vi "Cross With Speed Reference (1 Ch).vi"(8 "error in (no error)":errorcluster, 10 "Speed Profile (Positions [s])":sgl[](array[numeric]), 11 "Waveform":waveform(sgl)) -> (0 "error out":errorcluster, 3 "Cross phase [degrees]":cluster{"f0":dbl, "df":dbl, "phase":sgl[]})   [LabVIEW 2017, in "VibrationAnalysisFunctions.lvlib"]
uses:
  <vilib>/addons/InsightCM/Utilities/Analysis/Vibration/VibrationAnalysisFunctions.lvlib
  <vilib>/addons/_NISVFA/_Shared subVIs/Controls/svc_Window [Dual FFT].ctl
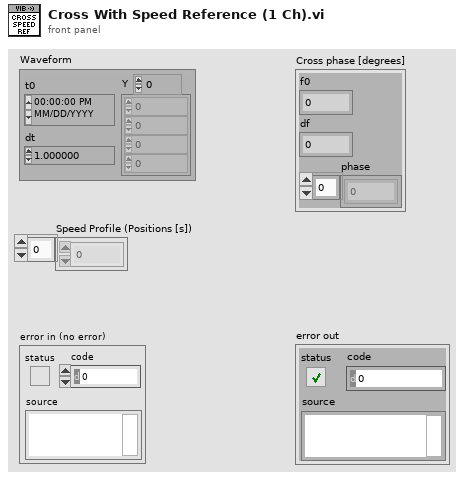
[diagram p1: front panel]
types:
  T1 = cluster{"dB On (T)":bool, "unwrap phase (F)":bool, "convert to degree (T)":bool}
  T2 = typedef "svc_Window [Dual FFT].ctl" = u32
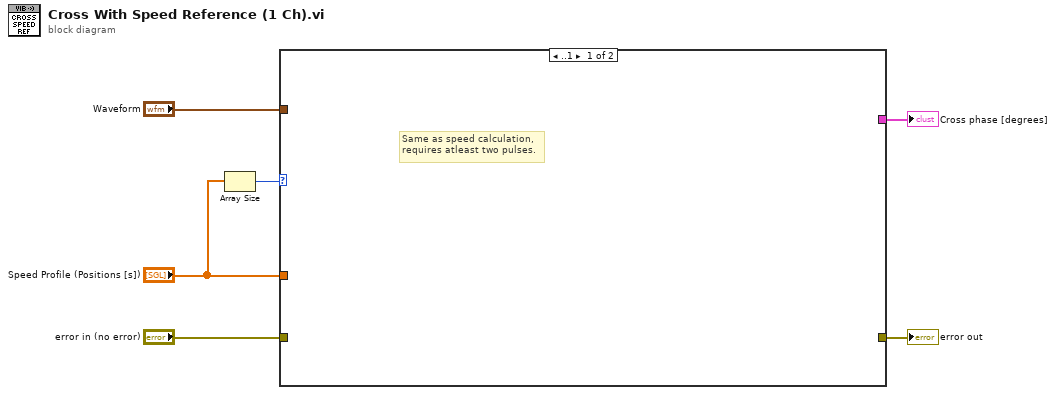
[diagram p0: block diagram]
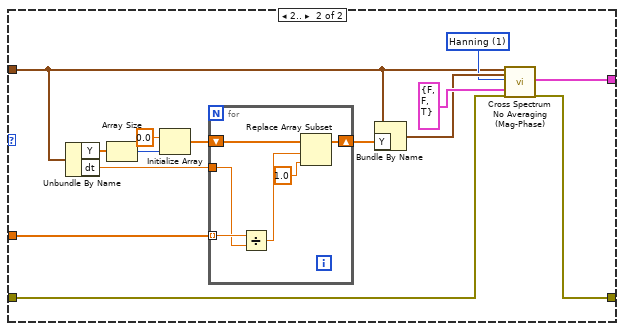
[diagram p2: hidden frame]
diagram:
  n1 = Array Size(array="Speed Profile (Positions [s])") -> (size(s)=w6:i32)
  n2 = case shown="..1" w6 {
    tunnel: "Waveform" -> [_ w7]
    tunnel: "Speed Profile (Positions [s])" -> [_ w8]
    tunnel: [_ w11] -> w3
    tunnel: [_ w9] -> w1
    tunnel: "error in (no error)" -> [_ w10]
    frame ..1 {
      # "Same as speed calculation,\nrequires atleast two pulses."
    }
    frame 2.. {
      w14 = T2 1 items=["None"=0, "Hanning"=1, "Hamming"=2, "Blackman-Harris"=3, "Exact Blackman"=4, "Blackman"=5, "Flat Top"=6, "4 Term B-Harris "=7, "7 Term B-Harris"=8, "Low Sidelobe"=9, "Force - Exponential"=10, "Blackman Nuttall"=11, "Triangle"=30, "Bartlett-Hanning"=31, "Bohman"=32, "Parzen"=33, "Welch"=34, "Kaiser"=60, "Dolph-Chebyshev"=61, "Gaussian"=62] ("window")
      n3 = Unbundle By Name(w7) -> ("Y"=w13:sgl[], "dt"=w12:dbl)
      n4 = Array Size(array=w13) -> (size(s)=w19:i32)
      n5 = Initialize Array(sgl 0.0 ("element"), w19) -> (w17:sgl[])
      n6 = for {
        shift-right: [w25] -> w16
        shift-left: w17 -> [w26]
        tunnel: w8 -> [w23] mode=indexing
        tunnel: w12 -> [w22]
        n7 = Divide(x=w23, y=w22) -> (x/y=w21:dbl)
        n8 = Replace Array Subset(array=w26, new element=sgl 1.0 ("new element/subarray"), index=w21) -> (w25:sgl[])
      }
      n9 = Bundle By Name(cluster=w7, "Y"=w16) -> (w15:waveform(sgl))
      n10 = call <vilib>:"Cross Spectrum No Averaging (Mag-Phase).vi"("scaled signal X [EUx]"=w7, "scaled signal Y [EUy]"=w15, "window"=w14, "view"=T1 {"dB On (T)"=FALSE, "unwrap phase (F)"=FALSE, "convert to degree (T)"=TRUE}, "error in (no error)"=w10) -> ("phase [degrees]"=w11:cluster{"f0":dbl, "df":dbl, "phase":sgl[]}, "error out"=w9:errorcluster)  [unwired: 12 in, 1 out]
    }
  }
  "Cross phase [degrees]" <- w3
  "error out" <- w1
